vi "M04 Hybrid car.vi"(9 "Angle in":sgl=-133.0, 11 "EV3 in":T1) -> (1 "Angle out":sgl, 3 "EV3 out":T1)   [LabVIEW 2016]
uses:
  <vilib>/NXT/Subs/LVHSConnector.ctl
  <vilib>/NXT/LegoClasses/BrickReference/BrickReference.lvclass
  <vilib>/NXT/Dual Mode Library/Waits/Wait_Num.vi
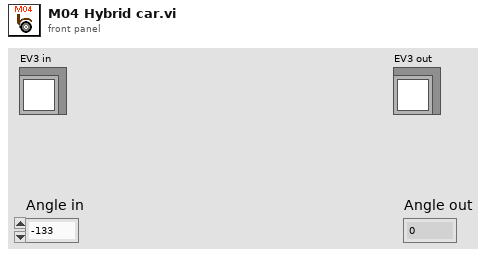
[diagram p1: front panel]
types:
  T1 = typedef "LVHSConnector.ctl" = refnum<class "BrickReference.lvclass">
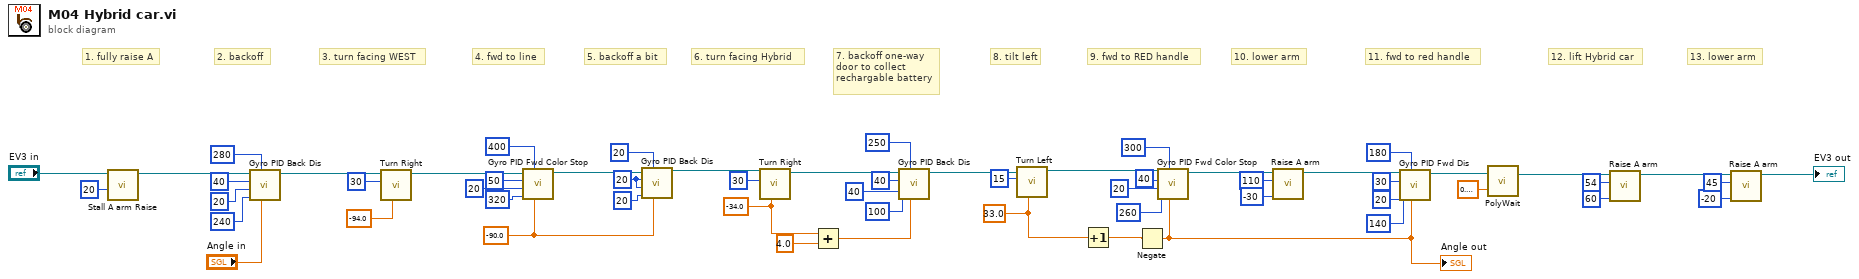
[diagram p0: block diagram]
diagram:
  w2 = sgl 33.0 ("Turning angle")
  w4 = 20 ("Max. speed")
  w48 = sgl -34.0 ("Turning angle")
  w27 = sgl -90.0 ("Target angle")
  # "8. tilt left"
  # "7. backoff one-way\ndoor to collect\nrechargable battery"
  # "2. backoff"
  # "1. fully raise A"
  # "5. backoff a bit"
  # "13. lower arm"
  # "12. lift Hybrid car"
  # "11. fwd to red handle"
  # "10. lower arm"
  # "9. fwd to RED handle"
  # "6. turn facing Hybrid"
  # "4. fwd to line"
  # "3. turn facing WEST"
  n1 = call "Stall A arm Raise.vi"("Power"=i8 20, "NXT/EV3"="EV3 in") -> ("NXT/EV3"=w11:T1)  [unwired: 9 in]
  n2 = call "Gyro PID Back Dis.vi"("Target angle"="Angle in", "Threshold to stop"=280, "Threshold to slow"=240, "Min. speed"=20, "Max. speed"=40, "EV3 in"=w11) -> ("EV3 out"=w10:T1)  [unwired: 5 in]
  n3 = call "Turn Right.vi"("Turning angle"=sgl -94.0, "Motor B (right)"=i8 30, "EV3 in"=w10) -> ("EV3 out"=w16:T1)  [unwired: 8 in]
  n4 = call "Gyro PID Fwd Color Stop.vi"("Target angle"=w27, "Threshold to Color"=400, "Threshold to slow"=320, "Min. speed"=20, "Max. speed"=50, "EV3 in"=w16) -> ("EV3 out"=w29:T1)  [unwired: 5 in]
  n5 = call "Gyro PID Back Dis.vi"("Target angle"=w27, "Threshold to stop"=20, "Threshold to slow"=20, "Min. speed"=w4, "Max. speed"=w4, "EV3 in"=w29) -> ("EV3 out"=w28:T1)  [unwired: 5 in]
  n6 = call "Turn Right.vi"("Turning angle"=w48, "Motor B (right)"=i8 30, "EV3 in"=w28) -> ("EV3 out"=w24:T1)  [unwired: 8 in]
  n7 = Add(x=w48, y=sgl 4.0) -> (x+y=w20:sgl)
  n8 = call "Gyro PID Back Dis.vi"("Target angle"=w20, "Threshold to stop"=250, "Threshold to slow"=100, "Min. speed"=40, "Max. speed"=40, "EV3 in"=w24) -> ("EV3 out"=w6:T1)  [unwired: 5 in]
  n9 = call "Turn Left.vi"("Turning angle"=w2, "Motor B (right)"=i8 15, "EV3 in"=w6) -> ("EV3 out"=w7:T1)  [unwired: 8 in]
  n10 = Increment(x=w2) -> (x+1=w1:sgl)
  n11 = Negate(x=w1) -> (-x=w5:sgl)
  "Angle out" <- w5
  n12 = call "Gyro PID Fwd Color Stop.vi"("Target angle"=w5, "Threshold to Color"=300 ("Stop rotation"), "Threshold to slow"=260 ("Threshold to De-acc"), "Min. speed"=20 ("Higher speed"), "Max. speed"=40 ("Acc"), "EV3 in"=w7) -> ("EV3 out"=w41:T1)  [unwired: 5 in]
  n13 = call "Raise A arm.vi"("Power"=i8 -30, "Rotation"=110, "EV3 in"=w41) -> ("EV3 out"=w38:T1)  [unwired: 8 in]
  n14 = call "Gyro PID Fwd Dis.vi"("Target angle"=w5, "Threshold to stop"=180, "Threshold to slow"=140, "Min. speed"=20, "Max. speed"=30, "EV3 in"=w38) -> ("EV3 out"=w35:T1)  [unwired: 5 in]
  n15 = call-poly <vilib>:"PolyWait.vi"("Time (1 sec)"=sgl 0.3, "NXT/EV3"=w35) -> ("NXT/EV3"=w3:T1)  [unwired: 2 in]
  n16 = call "Raise A arm.vi"("Power"=i8 60, "Rotation"=54, "EV3 in"=w3) -> ("EV3 out"=w31:T1)  [unwired: 8 in]
  n17 = call "Raise A arm.vi"("Power"=i8 -20, "Rotation"=45, "EV3 in"=w31) -> ("EV3 out"=→"EV3 out":T1)  [unwired: 8 in]
